vi "PulseTriggeredHist.vi"(10 "PMT in":bool[](array[boolean])=[FALSE, FALSE, FALSE, FALSE, FALSE, FALSE, FALSE, FALSE, FALSE, FALSE], 11 "Rising flank?":bool) -> (3 "HistoAdd out":u32[](array[numeric]))   [LabVIEW 2012]
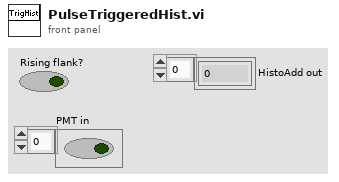
[diagram p1: front panel]
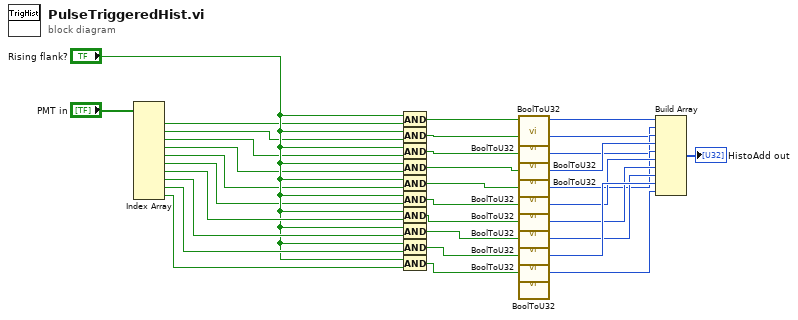
[diagram p0: block diagram]
diagram:
  n1 = Index Array(array="PMT in") -> (element #1=w2:bool, element #2=w3:bool, element #3=w4:bool, element #4=w5:bool, element #5=w6:bool, element #6=w7:bool, element #7=w9:bool, element #8=w10:bool, element #9=w11:bool, element #10=w12:bool)  [unwired: 10 in]
  n2 = And(x="Rising flank?", y=w2) -> (x .and. y?=w13:bool)
  n3 = And(x="Rising flank?", y=w3) -> (x .and. y?=w14:bool)
  n4 = And(x="Rising flank?", y=w4) -> (x .and. y?=w15:bool)
  n5 = And(x="Rising flank?", y=w5) -> (x .and. y?=w16:bool)
  n6 = And(x="Rising flank?", y=w6) -> (x .and. y?=w17:bool)
  n7 = And(x="Rising flank?", y=w7) -> (x .and. y?=w18:bool)
  n8 = And(x="Rising flank?", y=w9) -> (x .and. y?=w19:bool)
  n9 = And(x="Rising flank?", y=w10) -> (x .and. y?=w20:bool)
  n10 = And(x="Rising flank?", y=w11) -> (x .and. y?=w21:bool)
  n11 = And(x="Rising flank?", y=w12) -> (x .and. y?=w22:bool)
  n12 = call "BoolToU32.vi"("Boolean"=w13) -> ("Numeric"=w23:u32)  [unwired: 10 in]
  n13 = call "BoolToU32.vi"("Boolean"=w14) -> ("Numeric"=w24:u32)  [unwired: 10 in]
  n14 = call "BoolToU32.vi"("Boolean"=w15) -> ("Numeric"=w25:u32)  [unwired: 10 in]
  n15 = call "BoolToU32.vi"("Boolean"=w16) -> ("Numeric"=w26:u32)  [unwired: 10 in]
  n16 = call "BoolToU32.vi"("Boolean"=w17) -> ("Numeric"=w27:u32)  [unwired: 10 in]
  n17 = call "BoolToU32.vi"("Boolean"=w18) -> ("Numeric"=w28:u32)  [unwired: 10 in]
  n18 = call "BoolToU32.vi"("Boolean"=w19) -> ("Numeric"=w29:u32)  [unwired: 10 in]
  n19 = call "BoolToU32.vi"("Boolean"=w20) -> ("Numeric"=w30:u32)  [unwired: 10 in]
  n20 = call "BoolToU32.vi"("Boolean"=w21) -> ("Numeric"=w31:u32)  [unwired: 10 in]
  n21 = call "BoolToU32.vi"("Boolean"=w22) -> ("Numeric"=w32:u32)  [unwired: 10 in]
  n22 = Build Array(w23, w24, w25, w26, w27, w28, w29, w30, w31, w32) -> (→"HistoAdd out":u32[])
